vi "Addressing_shift_last_1.vi"(8 "error in (no error)":errorcluster, 11 "VALUE":u32=121 format="%08b") -> (0 "error out":errorcluster, 2 "Last Value":bool, 3 "Value >>1":u32 format="%08b")   [LabVIEW 2014, in "Driver_interaction.lvlib" / "Dali_usb_tridonics.lvclass"]
doc: "Shit the last 1, one position to the right.\nFor example:\n1100 0100 -> 1100 0010"
uses:
  Dali_usb_tridonics.lvclass
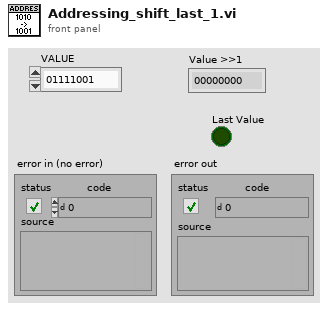
[diagram p1: front panel]
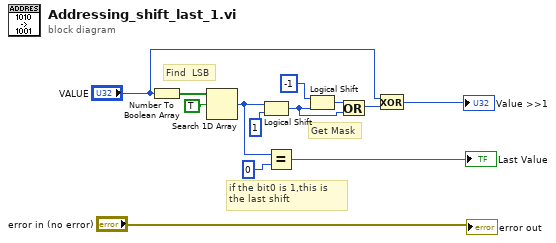
[diagram p0: block diagram]
diagram:
  # "Get Mask"
  # "if the bit0 is 1,this is the last shift"
  # "Find  LSB"
  n1 = Number To Boolean Array(number="VALUE") -> (Boolean array=w5:bool[])
  n2 = Search 1D Array(1D array=w5, element=TRUE) -> (index of element=w3:i32)  [unwired: 1 in]
  n3 = Logical Shift(y=w3, x=u32 1) -> (x << y=w10:u32)
  n4 = Equal?(x=w3, y=0) -> (x = y?=→"Last Value":bool)
  n5 = Logical Shift(y=i16 -1, x=w10) -> (x << y=w9:u32)
  n6 = Or(x=w9, y=w10) -> (x .or. y?=w11:u32)
  n7 = Exclusive Or(1:w11, 2:"VALUE") -> (0:→"Value >>1":u32)
  "error out" <- "error in (no error)"
